vi "_TextTestResult_Init.vi"(5 "testStartedEventRef":refnum<user-event>, 6 "verbosity":u32, 7 "resultStatusChangedEventRef":refnum<user-event>, 8 "error in (no error)":errorcluster, 9 "descriptions":bool, 10 "stream":refnum<queue>, 11 "TestTestResult in":refnum<class "_TextTestResult.lvclass">) -> (0 "error out":errorcluster, 3 "TestTestResult out":refnum<class "_TextTestResult.lvclass">)   [LabVIEW 2011, in "_TextTestResult.lvclass"]
uses:
  _TextTestResult.lvclass
  TestResult/resultStatusChanged--Cluster.ctl
  TestResult/resultStatus--enum.ctl
  TestResult/testStarted--Cluster.ctl
  _TextTestResult.lvclass/_TextTestResult.ctl
  TestResult/TestResult.lvclass
panel:
  # "JKI VI Tester for LabVIEW\nhttp://jkisoft.com/vi-tester\nCopyright (C) 2007-2009, JKI <info@jkisoft.com>\nALL RIGHTS RESERVED"
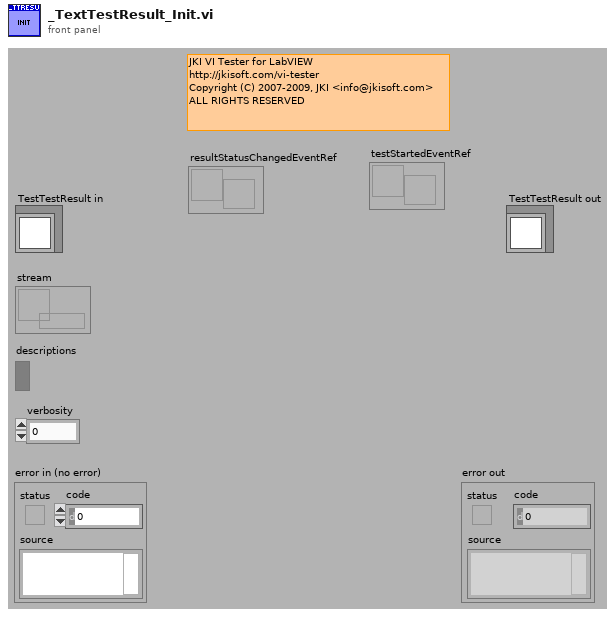
[diagram p1: front panel]
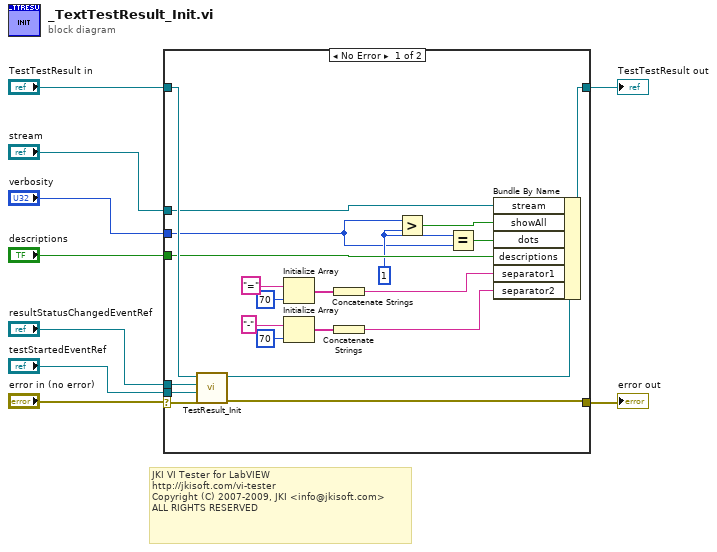
[diagram p0: block diagram]
diagram:
  # "JKI VI Tester for LabVIEW\nhttp://jkisoft.com/vi-tester\nCopyright (C) 2007-2009, JKI <info@jkisoft.com>\nALL RIGHTS RESERVED"
  n1 = case shown="No Error" "error in (no error)" {
    selector: "error in (no error)" -> [w29 w31]
    tunnel: "TestTestResult in" -> [w27 w32]
    tunnel: [w30 w32] -> w8
    tunnel: [w28 w31] -> w6
    tunnel: "descriptions" -> [w25 _]
    tunnel: "stream" -> [w24 _]
    tunnel: "verbosity" -> [w20 _]
    tunnel: "resultStatusChangedEventRef" -> [w11 _]
    tunnel: "testStartedEventRef" -> [w10 _]
    frame No Error {
      w21 = u32 1 ("y")
      n2 = call "TestResult_Init.vi"("error in (no error)"=w29, "testStartedEventRef"=w10, "resultStatusChangedEventRef"=w11, "TestResult in"=w27) -> ("error out"=w28:errorcluster, "TestResult out"=w26:refnum<class "_TextTestResult.lvclass">)  [unwired: 6 in]
      n3 = Initialize Array("=", 70 ("dimension size")) -> (w15:string[])
      n4 = Initialize Array("-", 70 ("dimension size")) -> (w13:string[])
      n5 = Concatenate Strings(w15) -> (w14:string)
      n6 = Concatenate Strings(w13) -> (w12:string)
      n7 = Greater?(x=w20, y=w21) -> (0:w23:bool)
      n8 = Equal?(x=w21, y=w20) -> (x = y?=w22:bool)
      n9 = Bundle By Name(cluster=w26, "stream"=w24, "showAll"=w23, "dots"=w22, "descriptions"=w25, "separator1"=w14, "separator2"=w12) -> (w30:refnum<class "_TextTestResult.lvclass">)
    }
    frame Error {
    }
  }
  "TestTestResult out" <- w8
  "error out" <- w6
